vi "Acquire.vi"(8 "error in (no error)":errorcluster, 10 "Msg in":T4, 11 "PXIDigitizer in":refnum<class "MagAnalysis_Online.lvclass">) -> (0 "error out":errorcluster, 1 "new command":string, 2 "Msg out":T4, 3 "PXIDigitizer out":refnum<class "MagAnalysis_Online.lvclass">)   [LabVIEW 2013, in "MagAnalysis_Online.lvclass"]
uses:
  MagAnalysis_Online.lvclass
  DriverMsg.ctl
  specInfo_TypDef.ctl
  userROI.ctl
  source/Device Driver/shared/numericVariable_TypeDef.ctl
  reshapeArrayCommand_TypDEf.ctl
  specClustercommandTypdef.ctl
  MagAnalysis_Online.lvclass/MagAnalysis_Online.ctl
  source/Device Driver/BaseDriver/BaseDriver.lvclass
panel:
  out "Array":bool[](array[boolean])
  out "Settings.CamSettings.Cam 0.UserROI":T1
  in  "B[T]MAIN":dbl
  out "image ok":bool[](array[boolean])
  out "time:FGV":u32
  out "time:updateSpec":u32
  out "time 2Dimage":u32
  out "time:specPost":u32
  out "time:div":u32
  out "time post":u32
  out "tima: aqu":u32
  out "offset":dbl
  out "post":dbl[][](array[numeric])
  out "new ROI":bool
  in  "increment":bool
  out "online":dbl[][](array[numeric])
  out "cHARGE":dbl[][](array[numeric])
  out "time 3":u32
  out "time 2":u32
  out "time 1":u32
  out "time 0":u32
  out "time all":u32
  out "time get images":u32
  out "B [T]":dbl
  out "specInfo":T3 {"Charge [pC]" format="%0.4f"}
  in  "Numeric":i32=95
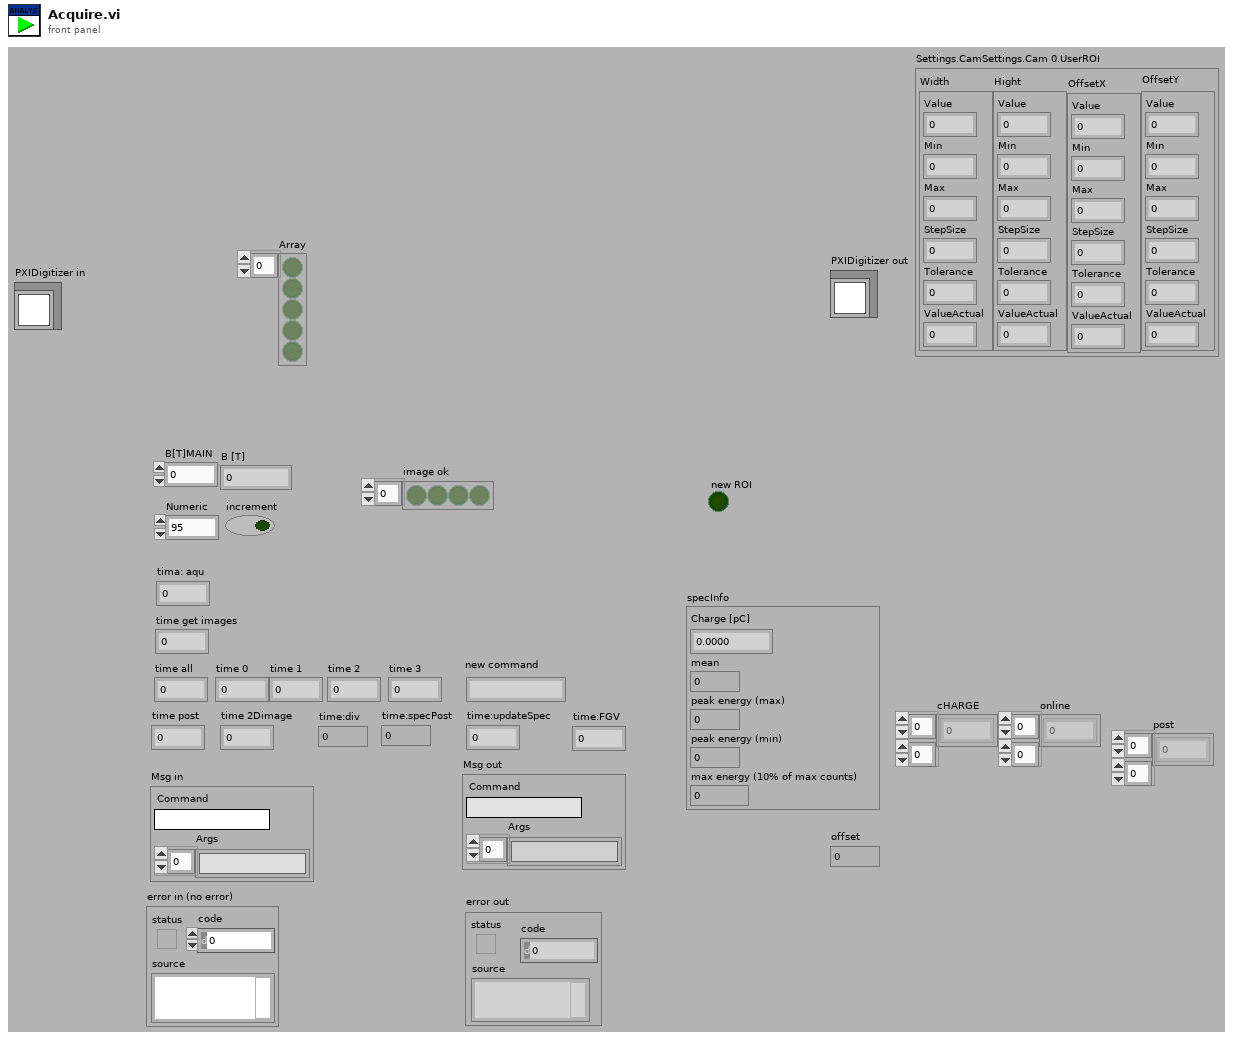
[diagram p1: front panel]
types:
  T1 = typedef "userROI.ctl" = cluster{"Width":T2, "Hight":T2, "OffsetX":T2, "OffsetY":T2}
  T2 = typedef "BaseDriver.lvclass/numericVariable_TypeDef.ctl" = cluster{"Value":dbl, "Min":dbl, "Max":dbl, "StepSize":dbl, "Tolerance":dbl, "ValueActual":dbl}
  T3 = typedef "specInfo_TypDef.ctl" = cluster{"Charge [pC]":dbl, "mean":dbl, "peak energy (max)":dbl, "peak energy (min)":dbl, "max energy (10% of max counts)":dbl}
  T4 = typedef "DriverMsg.ctl" = cluster{"Command":string, "Args":string[]}
  T5 = typedef "reshapeArrayCommand_TypDEf.ctl" = enum16{"init array", "addImage", "read", "init resolution"}
  T6 = typedef "specClustercommandTypdef.ctl" = enum16{"init", "addCluster", "read", "clear"}
  T7 = typedef "MagAnalysis_Online.lvclass/analysis_data_typdef.ctl" = cluster{"cam0":T8, "cam1":T8, "cam2":T8, "cam3":T8}
  T8 = typedef "IMAQ Image.ctl" = refnum<image>
  T9 = typedef "IMAQdx.ctl" = refnum<k21>
  T10 = typedef "bgImages_tyudef.ctl" = cluster{"cam 0":T8, "cam 1":T8, "cam 2":T8, "cam 3":T8}
  T11 = typedef "fileCluster_TypDef.ctl" = cluster{"spec cluster":cluster{dbl[], dbl[]}, "change from file":dbl, "B [T]":dbl, "spec cluster 2":cluster{dbl[], dbl[]}[]}
  T12 = typedef "OnOffTypeDef.ctl" = enum16{"off", "on"}
  T13 = typedef "Calib_Typdef.ctl" = cluster{"cam 0":T14, "cam 1":T14, "cam 2":T14, "cam 3":T14}
  T14 = typedef "calib_Sub_Typdef.ctl" = cluster{"incident ANGLE COMPENSATION":dbl[], "dp/B [MeV/C/B]":dbl[], "charge compensation":dbl[], "Momentum [MeV/C]":dbl[], "energyDependence Input":dbl[], "pixel angle (y)":dbl[], "dp [MeV/C/] ":dbl[], "angle 2Dfor spectrumj":dbl[][], "dp [MeV/C] 2D":dbl[][], "charge compensation 2D":dbl[][], "Screen&Camera 2":T15, "ROI info":T17, "Y 2D full angle":dbl[][], "calib pixel":T18, "2D":T19, "UserROI":T20, "final":T21, "B[T]":dbl, "index":dbl}
  T15 = typedef "ScreenCam2_TypDEf.ctl" = cluster{"Screen Orientation":string, "Screen angle":string, "Lens":T16, "Calibration (mm/pix)":dbl}
  T16 = typedef "CamAndObj_TypDEf.ctl" = enum16{"FL1-f8x08", "FL1-f8x06", "FL1-f8", "ch300-f50", "FL2G-f8", "FL3M14-f8", "FL3M14-f8x08", "FL3M14-f8x08(2x2)"}
  T17 = typedef "ROIInfo_TypDef.ctl" = cluster{"npix-X":i32, "npix-Y":i32, "Left [pix]":dbl, "Top [pix]":dbl}
  T18 = typedef "calibPixel.ctl" = cluster{"y1(pixel)":dbl[], "y2(pixel)":dbl[], "dp/B [MeV/C/B] (pixel)":dbl[], "energyDependence Input(pixel)":dbl[], "bending angle [deg](pixel)":dbl[], "total path(pixel)":dbl[], "pixel angle (y)(pixel)":dbl[], "energy dependence (pixel)":dbl[], "charge compensation (pixel)":dbl[], "Momentum [MeV/C](pixel)":dbl[], "angular compensation(pixel)":dbl[]}
  T19 = typedef "2DTypDef.ctl" = cluster{"dp":dbl[][], "chargeCompensation":dbl[][], "angle":dbl[][], "Momentum":dbl[][]}
  T20 = typedef "CamRoiTypDef.ctl" = cluster{"Width":dbl, "Hight":dbl, "OffsetX":dbl, "OffsetY":dbl}
  T21 = typedef "finalCalibTypdef.ctl" = cluster{"X":dbl[][], "xi":dbl[][], "delta momentum":dbl, "Y":dbl[][], "yi":dbl[][], "angle (Y)":dbl[], "delta angle":dbl, "scale delta angle":dbl, "intraX":dbl, "intraY":dbl, "mask":dbl[][]}
  T22 = typedef "specCluster_Typdef.ctl" = cluster{"dp [MeV/C]":dbl[], dbl[]}
  T23 = typedef "reshapeINfo_TypDef.ctl" = cluster{"emptyImageArray":dbl[], "max Y size":i32, "X size":i32, "number of cam":i32, "emptyZArrayforreshape":T24}
  T24 = typedef "emptyArray_TYpDEf.ctl" = cluster{"Cam 0":T25, "Cam 1":T25, "Cam 2":T25, "Cam 3":T25}
  T25 = typedef "emptyArrayCamX_TypDef.ctl" = cluster{"1":dbl[][], "2":dbl[][]}
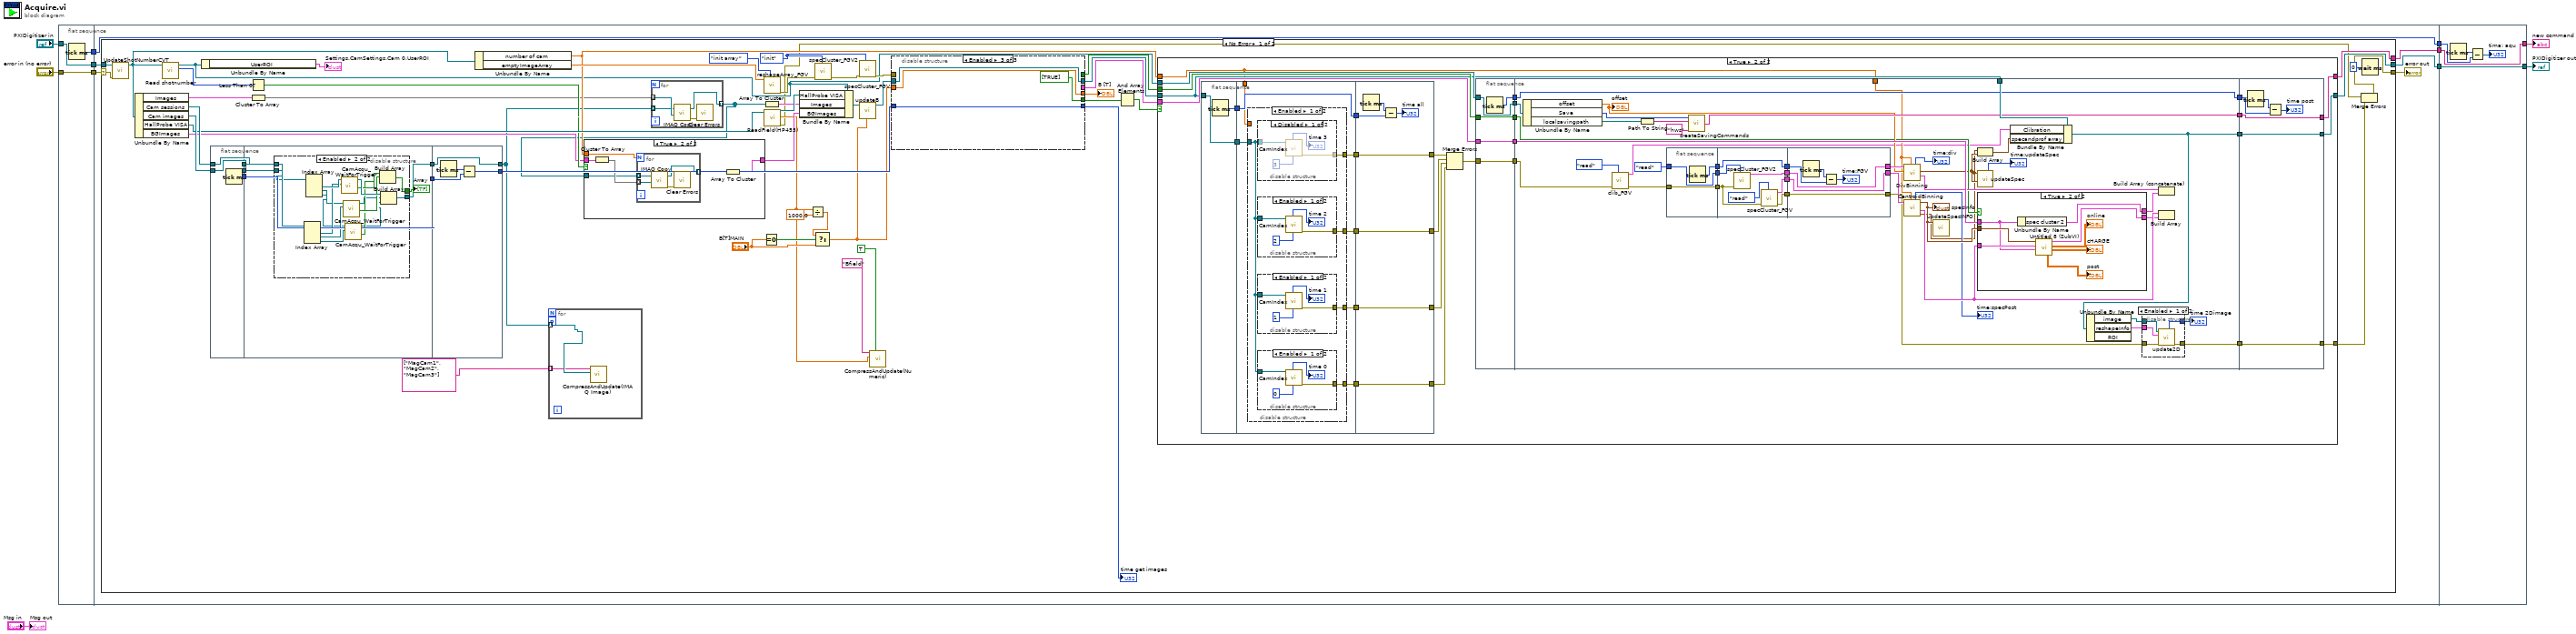
[diagram p0: block diagram]
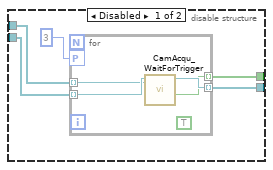
[diagram p2: hidden frame]
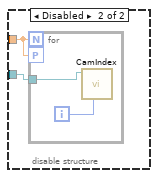
[diagram p11: hidden frame]
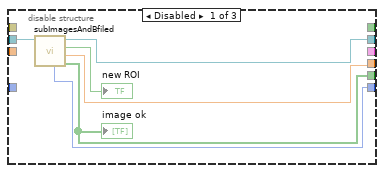
[diagram p12: hidden frame]
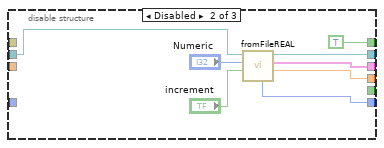
[diagram p13: hidden frame]
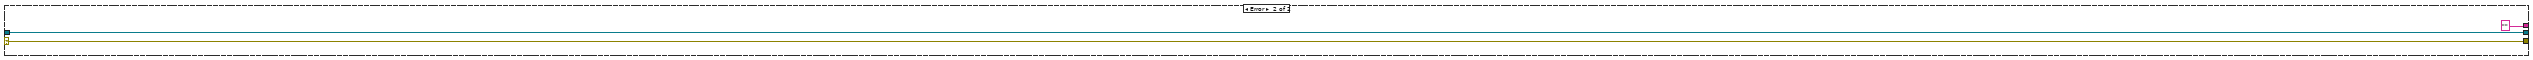
[diagram p14: hidden frame]
diagram:
  n1 = flat-sequence {
    tunnel: "error in (no error)" -> [w13]
    tunnel: "PXIDigitizer in" -> [w14]
    tunnel: [w14] -> w4
    tunnel: [w13] -> w3
    tunnel: [w12] -> w2
    tunnel: [w20] -> w6
    tunnel: [w16] -> w5
    tunnel: w4 -> [w19]
    tunnel: w3 -> [w17]
    tunnel: w2 -> [w15]
    tunnel: [w15] -> w1
    tunnel: [w309] -> w7
    tunnel: [w310] -> w11
    tunnel: w6 -> [w310]
    tunnel: w5 -> [w309]
    tunnel: w1 -> [w307]
    frame #0 {
      n2 = Tick Count (ms)() -> (millisecond timer value=w12:u32)
    }
    frame #1 {
      n3 = case shown="No Error" w17 {
        selector: w17 -> [w75 w304]
        tunnel: w19 -> [w74 w305]
        tunnel: [w67 w305] -> w20
        tunnel: [w22 w304] -> w18
        tunnel: [w65 "" ("new command")] -> w16
        frame No Error {
          w62 = specClustercommandTypdef."init" ("command")
          n4 = call "UpdateShotNumberCVT.vi"("error in (no error)"=w75, "BaseDriver in"=w74) -> ("BaseDriver out"=w52:refnum<class "MagAnalysis_Online.lvclass">)  [unwired: 8 in, 1 out]
          n5 = Unbundle By Name(w52) -> ("Images"=w34:T7, "Cam sessions"=w57:T9[], "Cam images"=w56:T8[], "HallProbe VISA"=w55:refnum<visa-resource-name>, "BGImages"=w49:T10)
          n6 = call-dynamic "Read shotnumber.vi"("BaseDriver in"=w52) -> ("shotnumber"=w51:i32, "BaseDriver out"=w39:refnum<class "MagAnalysis_Online.lvclass">)  [unwired: 7 in, 2 out]
          n7 = Unbundle By Name(w39) -> ("UserROI"=→"Settings.CamSettings.Cam 0.UserROI":T1)
          n8 = flat-sequence {
            tunnel: w56 -> [w83]
            tunnel: w57 -> [w84]
            tunnel: [w84] -> w45
            tunnel: [w83] -> w44
            tunnel: [w82] -> w43
            tunnel: [w87] -> w46
            tunnel: w45 -> [w89]
            tunnel: w44 -> [w88]
            tunnel: w43 -> [w86]
            tunnel: [w86] -> w42
            tunnel: [w118] -> w30
            tunnel: w46 -> [w118]
            tunnel: w42 -> [w116]
            tunnel: [w115] -> w41
            frame #0 {
              n9 = Tick Count (ms)() -> (millisecond timer value=w82:u32)
            }
            frame #1 {
              n10 = disable-structure shown="Enabled" {
                disable-tunnel: w89 -> [w91 w114]
                disable-tunnel: w88 -> [w94 w113]
                disable-tunnel: [w93 w109] -> w87
                disable-tunnel: [w92 w99] -> w85
                frame Disabled {
                  n11 = for {
                    tunnel: w91 -> [w97] mode=indexing
                    tunnel: w94 -> [w98] mode=indexing
                    tunnel: [w96] -> w93 mode=indexing
                    workers-P: 3 -> [_]
                    tunnel: [w95] -> w92 mode=indexing
                    (unwired) TRUE ("cam conneced")
                    n12 = call "CamAcqu_WaitForTrigger.vi"("Session in"=w97, "Image in"=w98) -> ("Acquisition OK?"=w95:bool, "Image  Out"=w96:T8)  [unwired: 7 in, 1 out]
                  }
                }
                frame Enabled {
                  n13 = Index Array(array=w114) -> (element #1=w111:T9, element #2=w106:T9, element #3=w104:T9)  [unwired: 3 in]
                  n14 = Index Array(array=w113) -> (element #1=w112:T8, element #2=w107:T8, element #3=w105:T8)  [unwired: 3 in]
                  n15 = call "CamAcqu_WaitForTrigger.vi"("Session in"=w111, "Image in"=w112) -> ("Acquisition OK?"=w108:bool, "Image  Out"=w110:T8)  [unwired: 7 in, 1 out]
                  n16 = call "CamAcqu_WaitForTrigger.vi"("Session in"=w106, "Image in"=w107) -> ("Acquisition OK?"=w103:bool, "Image  Out"=w101:T8)  [unwired: 7 in, 1 out]
                  n17 = call "CamAcqu_WaitForTrigger.vi"("Session in"=w104, "Image in"=w105) -> ("Acquisition OK?"=w102:bool, "Image  Out"=w100:T8)  [unwired: 7 in, 1 out]
                  n18 = Build Array(w108, w103, w102) -> (w99:bool[])
                  n19 = Build Array(w110, w101, w100) -> (w109:T8[])
                }
              }
              "Array" <- w85
            }
            frame #2 {
              n20 = Tick Count (ms)() -> (millisecond timer value=w117:u32)
              n21 = Subtract(x=w117, y=w116) -> (x-y=w115:u32)
            }
          }
          n22 = Less Than 0?(x=w51) -> (x < 0?=w50:bool)
          n23 = Cluster To Array(cluster=w34) -> (array=w32:T8[])
          n24 = Unbundle By Name(w52) -> ("number of cam"=w48:dbl, "emptyImageArray"=w73:dbl[])
          n25 = for {
            tunnel: w30 -> [w77] mode=indexing
            tunnel: string[] ["MagCam1", "MagCam2", "MagCam3"] -> [w76] mode=indexing
            workers-P: _ -> [_]
            n26 = call "CompressAndUpdate(IMAQ Image).vi"("IMAQ Image"=w77, "command or variable name"=w76) -> ()  [unwired: 9 in, 1 out]
          }
          n27 = for {
            tunnel: w32 -> [w81] mode=indexing
            tunnel: w30 -> [w80] mode=indexing
            tunnel: [w79] -> w31 mode=indexing
            n28 = call "IMAQ Copy"("Image Dst"=w81, "Image Src"=w80) -> ("error out"=w78:errorcluster, "Image Dst Out"=w79:T8)  [unwired: 4 in]
            n29 = call "Clear Errors.vi"("error in (no error)"=w78) -> ()  [unwired: 6 in, 1 out]
          }
          n30 = case shown="True" w50 {
            tunnel: [w119 w122] -> w47
            tunnel: w49 -> [w119 w125]
            tunnel: w48 -> [_ w121]
            tunnel: w31 -> [_ w120]
            frame False {
            }
            frame True {
              n31 = Cluster To Array(cluster=w125) -> (array=w124:T8[])
              n32 = for {
                N: w121 -> [_]
                tunnel: w124 -> [w129] mode=indexing
                tunnel: w120 -> [w128] mode=indexing
                tunnel: [w127] -> w123 mode=indexing
                n33 = call "IMAQ Copy"("Image Dst"=w129, "Image Src"=w128) -> ("error out"=w126:errorcluster, "Image Dst Out"=w127:T8)  [unwired: 4 in]
                n34 = call "Clear Errors.vi"("error in (no error)"=w126) -> ()  [unwired: 6 in, 1 out]
              }
              n35 = Array To Cluster(array=w123) -> (cluster=w122:cluster{"[0]":T8, "[1]":T8, "[2]":T8, "[3]":T8})
            }
          }
          n36 = Array To Cluster(array=w31) -> (cluster=w33:cluster{"[0]":T8, "[1]":T8, "[2]":T8, "[3]":T8})
          n37 = Equal To 0?(x="B[T]MAIN") -> (x = 0?=w36:bool)
          n38 = call "reshapeArray_FGV.vi"("command"=reshapeArrayCommand_TypDEf."init array", "emptyImageArray"=w73) -> ("error in (no error) 2"=w64:errorcluster)  [unwired: 8 in, 1 out]
          n39 = call "ReadField(HP455).vi"("VISA Refnum in"=w55) -> ("error out"=w21:errorcluster, "B-Field [mT]"=w25:dbl, "VISA resource name out"=w53:refnum<visa-resource-name>)  [unwired: 8 in]
          n40 = Bundle By Name(cluster=w39, "HallProbe VISA"=w53, "Images"=w33, "BGImages"=w47) -> (w38:refnum<class "MagAnalysis_Online.lvclass">)
          n41 = Divide(x=w25, y=1000.0) -> (x/y=w23:dbl)
          n42 = Select(t=w23, s=w36, f="B[T]MAIN") -> (s? t:f=w28:dbl)
          n43 = call "specCluster_FGV2.vi"("command"=w62, "error in (no error)"=w64) -> ("error out"=w63:errorcluster)  [unwired: 8 in, 1 out]
          n44 = call "specCluster_FGV.vi"("command"=w62, "error in (no error)"=w63) -> ("error out"=w71:errorcluster)  [unwired: 8 in, 1 out]
          n45 = call "updateB.vi"("B [T] new"=w28, "MagAnalysis_Online in"=w38) -> ("MagAnalysis_Online out"=w37:refnum<class "MagAnalysis_Online.lvclass">)  [unwired: 9 in]
          n46 = call "CompressAndUpdate(Numeric).vi"("force CVT update (false)"=TRUE, "Numeric"=w25, "command or variable name"="Bfield") -> ()  [unwired: 8 in, 1 out]
          n47 = disable-structure shown="Enabled" {
            disable-tunnel: w71 -> [_ _ _]
            disable-tunnel: [w290 w298 w299] -> w70
            disable-tunnel: [w289 w297 w302] -> w58
            disable-tunnel: [w288 w292 w301] -> w54
            disable-tunnel: w37 -> [w287 w294 w302]
            disable-tunnel: [_ w293 _] -> w69
            disable-tunnel: [_ TRUE _] -> w68
            disable-tunnel: [w284 _ bool[] [TRUE] ("image ok")] -> w60
            disable-tunnel: w28 -> [_ _ w301]
            disable-tunnel: w41 -> [_ _ w299]
            frame Disabled {
              n48 = call "subImagesAndBfiled.vi"("MagAnalysis_Online in"=w287) -> ("image ok"=w284:bool[], "B[T]"=w288:dbl, "new ROI"=→"new ROI":bool, "MagAnalysis_Online out"=w289:refnum<class "MagAnalysis_Online.lvclass">, "Numeric 2"=w290:u32, "OK"=w285:bool[])  [unwired: 5 in]
              "image ok" <- w284
            }
            frame Disabled {
              n49 = call "fromFileREAL.vi"("increment"="increment", "Numeric"="Numeric", "MagAnalysis_Online in"=w294) -> ("B [T]"=w292:dbl, "Cluster"=w293:T11, "MagAnalysis_Online out"=w297:refnum<class "MagAnalysis_Online.lvclass">, "time"=w298:u32)  [unwired: 5 in]
            }
            frame Enabled {
            }
          }
          "B [T]" <- w54
          "time get images" <- w70
          n50 = And Array Elements(Boolean array=w60) -> (logical AND=w59:bool)
          n51 = case shown="True" w59 {
            tunnel: w69 -> [_ w138]
            tunnel: w68 -> [_ w137]
            tunnel: [w130 w136] -> w67
            tunnel: [_ w135] -> w66
            tunnel: w39 -> [_ w134]
            tunnel: [_ w133] -> w65
            tunnel: w58 -> [w130 w132]
            tunnel: w48 -> [_ w131]
            frame False {
            }
            frame True {
              n52 = flat-sequence {
                tunnel: w132 -> [w244]
                tunnel: [w244] -> w159
                tunnel: [w243] -> w158
                tunnel: w159 -> [w247]
                tunnel: [w251] -> w157
                tunnel: [w250] -> w156
                tunnel: [w249] -> w155
                tunnel: [w248] -> w154
                tunnel: w158 -> [w246]
                tunnel: [w246] -> w153
                tunnel: w131 -> [w245]
                tunnel: [w280] -> w140
                tunnel: [w281] -> w141
                tunnel: [w282] -> w142
                tunnel: [w283] -> w143
                tunnel: w157 -> [w283]
                tunnel: w156 -> [w282]
                tunnel: w155 -> [w281]
                tunnel: w154 -> [w280]
                tunnel: w153 -> [w278]
                frame #0 {
                  n53 = Tick Count (ms)() -> (millisecond timer value=w243:u32)
                }
                frame #1 {
                  n54 = disable-structure shown="Enabled" {
                    disable-tunnel: [w256 _] -> w251
                    disable-tunnel: [w255 _] -> w250
                    disable-tunnel: [w254 _] -> w249
                    disable-tunnel: [w253 _] -> w248
                    disable-tunnel: w247 -> [w252 w274]
                    disable-tunnel: w245 -> [_ w273]
                    frame Enabled {
                      n55 = disable-structure shown="Disabled" {
                        disable-tunnel: [w268 _] -> w256
                        disable-tunnel: w252 -> [w267 _]
                        frame Disabled {
                          n56 = call "CamIndex.vi"("index"=3, "MagAnalysis_Online in"=w267) -> ("error out"=w268:errorcluster, "time"=→"time 3":u32)  [unwired: 5 in, 3 out]
                        }
                        frame Enabled {
                        }
                      }
                      n57 = disable-structure shown="Enabled" {
                        disable-tunnel: [w260 _] -> w255
                        disable-tunnel: w252 -> [w259 _]
                        frame Enabled {
                          n58 = call "CamIndex.vi"("index"=2, "MagAnalysis_Online in"=w259) -> ("error out"=w260:errorcluster, "time"=→"time 2":u32)  [unwired: 5 in, 3 out]
                        }
                        frame Disabled {
                        }
                      }
                      n59 = disable-structure shown="Enabled" {
                        disable-tunnel: [w264 _] -> w254
                        disable-tunnel: w252 -> [w263 _]
                        frame Enabled {
                          n60 = call "CamIndex.vi"("index"=1, "MagAnalysis_Online in"=w263) -> ("error out"=w264:errorcluster, "time"=→"time 1":u32)  [unwired: 5 in, 3 out]
                        }
                        frame Disabled {
                        }
                      }
                      n61 = disable-structure shown="Enabled" {
                        disable-tunnel: [w272 _] -> w253
                        disable-tunnel: w252 -> [w271 _]
                        frame Enabled {
                          n62 = call "CamIndex.vi"("index"=0, "MagAnalysis_Online in"=w271) -> ("error out"=w272:errorcluster, "time"=→"time 0":u32)  [unwired: 5 in, 3 out]
                        }
                        frame Disabled {
                        }
                      }
                    }
                    frame Disabled {
                      n63 = for {
                        N: w273 -> [_]
                        workers-P: w273 -> [_]
                        tunnel: w274 -> [w275]
                        i -> [w276]
                        n64 = call "CamIndex.vi"("index"=w276, "MagAnalysis_Online in"=w275) -> ()  [unwired: 5 in, 5 out]
                      }
                    }
                  }
                }
                frame #2 {
                  n65 = Tick Count (ms)() -> (millisecond timer value=w279:u32)
                  n66 = Subtract(x=w279, y=w278) -> (x-y=→"time all":u32)
                }
              }
              n67 = Merge Errors(w143, w142, w141, w140) -> (w139:errorcluster)
              n68 = flat-sequence {
                tunnel: w134 -> [w161]
                tunnel: w137 -> [w162]
                tunnel: w138 -> [w163]
                tunnel: w139 -> [w164]
                tunnel: [w164] -> w152
                tunnel: [w163] -> w151
                tunnel: [w162] -> w150
                tunnel: [w161] -> w149
                tunnel: [w160] -> w148
                tunnel: w132 -> [w200]
                tunnel: [w197] -> w147
                tunnel: [w196] -> w146
                tunnel: [w190] -> w145
                tunnel: w152 -> [w205]
                tunnel: w151 -> [w202]
                tunnel: w150 -> [w178]
                tunnel: w149 -> [w192]
                tunnel: w148 -> [w183]
                tunnel: [w183] -> w144
                tunnel: w131 -> [w169]
                tunnel: [w240] -> w133
                tunnel: [w241] -> w135
                tunnel: [w242] -> w136
                tunnel: w147 -> [w242]
                tunnel: w146 -> [w241]
                tunnel: w145 -> [w240]
                tunnel: w144 -> [w238]
                frame #0 {
                  n69 = Tick Count (ms)() -> (millisecond timer value=w160:u32)
                }
                frame #1 {
                  n70 = Unbundle By Name(w192) -> ("offset"=w184:dbl, "Save"=w191:T12, "localsavingpath"=w193:path)
                  "offset" <- w184
                  n71 = call "clib_FGV.vi"("command"=specClustercommandTypdef."read", "error in (no error)"=w205) -> ("error out"=w171:errorcluster, "Clibration 2"=w165:T13)  [unwired: 8 in]
                  n72 = Path To String(path=w193) -> (string=w194:string)
                  n73 = flat-sequence {
                    tunnel: specClustercommandTypdef."read" ("command") -> [w215]
                    tunnel: [w215] -> w174
                    tunnel: [w214] -> w173
                    tunnel: w171 -> [w213]
                    tunnel: [w213] -> w170
                    tunnel: [w221] -> w177
                    tunnel: [w220] -> w176
                    tunnel: [w218] -> w175
                    tunnel: w174 -> [w219]
                    tunnel: w173 -> [w217]
                    tunnel: [w217] -> w172
                    tunnel: w170 -> [w216]
                    tunnel: [w226] -> w186
                    tunnel: [w227] -> w188
                    tunnel: [w228] -> w207
                    tunnel: w177 -> [w228]
                    tunnel: w176 -> [w227]
                    tunnel: w175 -> [w226]
                    tunnel: w172 -> [w224]
                    frame #0 {
                      n74 = Tick Count (ms)() -> (millisecond timer value=w214:u32)
                    }
                    frame #1 {
                      n75 = call "specCluster_FGV2.vi"("command"=w219, "error in (no error)"=w216) -> ("specArray"=w218:T22[])  [unwired: 8 in, 1 out]
                      n76 = call "specCluster_FGV.vi"("command"=specClustercommandTypdef."read", "error in (no error)"=w216) -> ("error out"=w220:errorcluster, "specArray"=w221:T22[])  [unwired: 8 in]
                    }
                    frame #2 {
                      n77 = Tick Count (ms)() -> (millisecond timer value=w225:u32)
                      n78 = Subtract(x=w225, y=w224) -> (x-y=→"time:FGV":u32)
                    }
                  }
                  n79 = call "createSavingCommands.vi"("extension"="hws" ("Fileextension"), "Saving Path (local)"=w194, "Save"=w191) -> ("String"=w190:string)  [unwired: 1 in]
                  n80 = call "DivBinning.vi"("Settings.number of cam"=w169, "offset"=w184, "spec cluster 3"=w186) -> ("spec cluster"=w185:cluster{"dp [MeV/C]":dbl[], dbl[]}, "divergence"=w168:waveform(dbl), "time:div"=→"time:div":u32)  [unwired: 6 in]
                  n81 = call "CentroidBinning.vi"("Settings.number of cam"=w169, "spec cluster 3"=w207) -> ("spectrum"=w167:waveform(dbl), "spec cluster"=w203:cluster{"xi used":dbl[], "yi":dbl[]}, "specInfo"=w204:T3, "time:specPost"=→"time:specPost":u32)  [unwired: 5 in, 1 out]
                  "specInfo" <- w204
                  n82 = call "updateSpecINFO.vi"("specInfo"=w204) -> ()  [unwired: 11 in]
                  n83 = Build Array(w167, w168) -> (w166:waveform(dbl)[])
                  n84 = call "updateSpec.vi"("profile"=w168, "spectrum"=w167) -> ("time:updateSpec"=→"time:updateSpec":u32)  [unwired: 9 in]
                  n85 = case shown="True" w178 {
                    tunnel: w204 -> [_ w236]
                    tunnel: w203 -> [_ w235]
                    tunnel: w202 -> [_ w230]
                    tunnel: [_ w234] -> w201
                    tunnel: [_ w229] -> w189
                    frame False {
                    }
                    frame True {
                      n86 = Unbundle By Name(w230) -> ("spec cluster 2"=w229:cluster{dbl[], dbl[]}[])
                      n87 = call "Untitled 8 (SubVI).vi"("Cluster 2"=w230, "spec cluster in"=w235, "specInfo"=w236) -> ("cHARGE"=→"cHARGE":dbl[][], "online"=→"online":dbl[][], "spec cluster out"=w234:cluster{dbl[], dbl[]}, "post"=→"post":dbl[][])  [unwired: 5 in]
                    }
                  }
                  n88 = Bundle By Name(cluster=w200, "Clibration"=w165, "specandprof array"=w166) -> (w197:refnum<class "MagAnalysis_Online.lvclass">)
                  n89 = Unbundle By Name(w197) -> ("image"=w199:T8, "reshapeInfo"=w198:T23)  [unwired: 1 out]
                  n90 = disable-structure shown="Enabled" {
                    disable-tunnel: w199 -> [w212 _]
                    disable-tunnel: w198 -> [w211 _]
                    disable-tunnel: [w210 _] -> w196
                    disable-tunnel: w188 -> [w209 _]
                    disable-tunnel: [w208 _] -> w180
                    frame Enabled {
                      n91 = call "update2D.vi"("error in (no error)"=w209, "reshapeInfo"=w211, "Image in"=w212) -> ("error out"=w210:errorcluster, "time 2Dimage"=w208:u32)  [unwired: 6 in, 1 out]
                    }
                    frame Disabled {
                    }
                  }
                  "time 2Dimage" <- w180
                  n92 = Build Array (concatenate)(w185, w189) -> ()  [unwired: 1 out]
                  n93 = Build Array(w203, w201) -> ()  [unwired: 1 out]
                }
                frame #2 {
                  n94 = Tick Count (ms)() -> (millisecond timer value=w239:u32)
                  n95 = Subtract(x=w239, y=w238) -> (x-y=→"time post":u32)
                }
              }
            }
          }
          n96 = Merge Errors(w21, w66) -> (w22:errorcluster)
          n97 = Wait (ms)(milliseconds to wait=u32 0) -> ()  [unwired: 1 out]
        }
        frame Error {
        }
      }
      "error out" <- w18
    }
    frame #2 {
      n98 = Tick Count (ms)() -> (millisecond timer value=w308:u32)
      n99 = Subtract(x=w308, y=w307) -> (x-y=→"tima: aqu":u32)
    }
  }
  "PXIDigitizer out" <- w11
  "new command" <- w7
  "Msg out" <- "Msg in"
